vi "Draw.vi"(7 "menu in":refnum<class "menu.lvclass">, 8 "error in (no error)":errorcluster, 11 "text item in":refnum<class "text item.lvclass">) -> (0 "error out":errorcluster, 3 "text item out":refnum<class "text item.lvclass">)   [LabVIEW 2009, in "text item.lvclass"]
uses:
  text item.lvclass
  Menu/menu.lvclass
  text item.lvclass/text item.ctl
  ICON/icon.lvclass
  Text/text.lvclass
  Menu Item/menu item.lvclass
  Arrow/arrow.lvclass
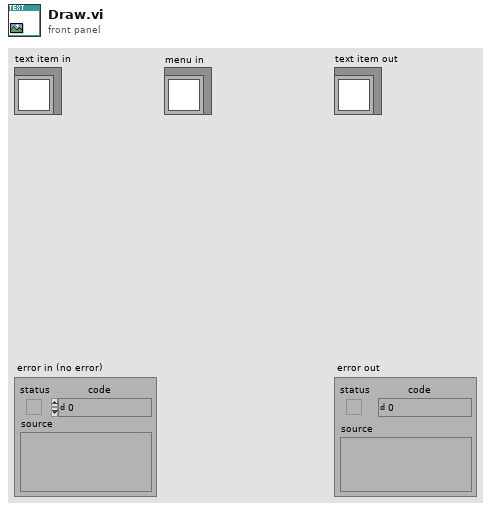
[diagram p1: front panel]
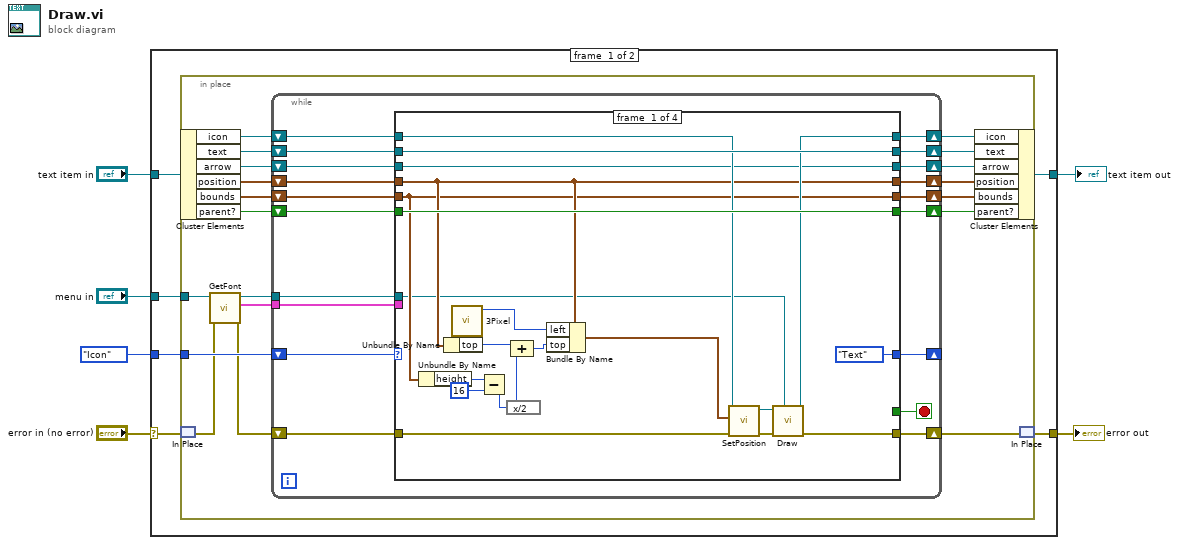
[diagram p0: block diagram]
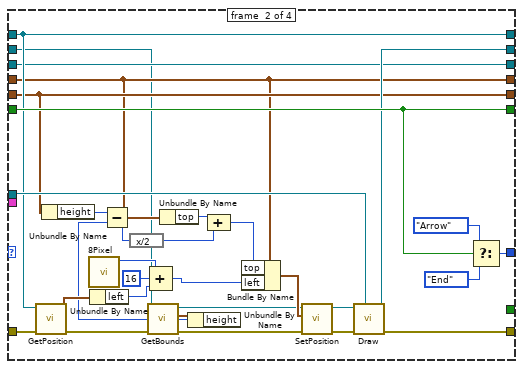
[diagram p2: hidden frame]
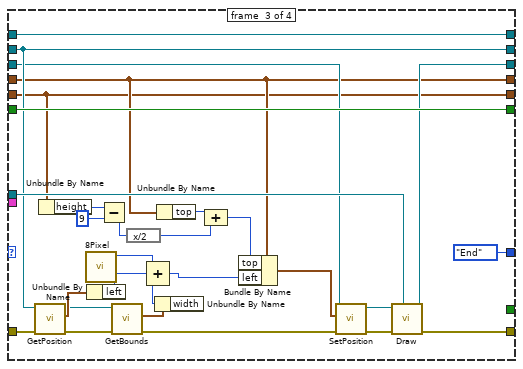
[diagram p3: hidden frame]
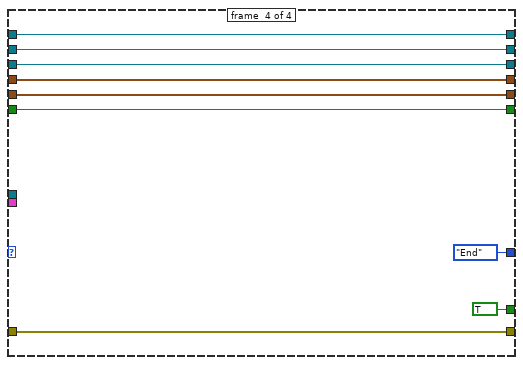
[diagram p4: hidden frame]
diagram:
  n1 = case shown="No Error" "error in (no error)" {
    selector: "error in (no error)" -> [w11 w142]
    tunnel: "text item in" -> [w12 w141]
    tunnel: [w10 w142] -> w4
    tunnel: [w9 w141] -> w3
    tunnel: "menu in" -> [w8 _]
    tunnel: enum16{"Icon", "Text", "Arrow", "End"}."Icon" -> [w7 _]
    frame #0 {
      n2 = in-place {
        in-place-border: w8 -> [w22]
        in-place-border: w7 -> [w31]
        n3 = in-place-cluster #1(w12) -> ("icon"=w30:refnum<class "icon.lvclass">, "text"=w29:refnum<class "text.lvclass">, "arrow"=w14:refnum<class "arrow.lvclass">, "position"=w28:cluster{"left":u32, "top":u32}, "bounds"=w27:cluster{"width":u32, "height":u32}, "parent?"=w16:bool)
        n4 = in-place-match #2(w11) -> (w20:errorcluster)
        n5 = call "GetFont.vi"("error in (no error)"=w20, "menu in"=w22) -> ("error out"=w19:errorcluster, "font"=w18:cluster{"name":string, "size":i16, "color":u32}, "menu out"=w21:refnum<class "menu.lvclass">)  [unwired: 7 in]
        n6 = while {
          shift-right: [w38] -> _
          shift-left: w31 -> [w50]
          shift-right: [w40] -> w17
          shift-left: w19 -> [w49]
          shift-right: [w41] -> w23
          shift-left: w27 -> [w45]
          shift-right: [w42] -> w24
          shift-left: w28 -> [w46]
          shift-right: [w43] -> w25
          shift-left: w29 -> [w47]
          shift-right: [w44] -> w26
          shift-left: w30 -> [w48]
          tunnel: w21 -> [w34]
          tunnel: w18 -> [w39]
          shift-right: [w37] -> w15
          shift-left: w16 -> [w36]
          shift-right: [w32] -> w13
          shift-left: w14 -> [w33]
          stop <- w35 stop-if-true
          n7 = case shown="\"Icon\"" w50 {
            tunnel: w49 -> [w66 w92 w125 w135]
            tunnel: w48 -> [w64 w93 w130 w140]
            tunnel: w47 -> [w70 w74 w124 w139]
            tunnel: w46 -> [w61 w82 w110 w138]
            tunnel: w45 -> [w60 w85 w109 w137]
            tunnel: [w63 w93 w130 w140] -> w44
            tunnel: [w70 w94 w124 w139] -> w43
            tunnel: [w61 w82 w110 w138] -> w42
            tunnel: [w60 w85 w109 w137] -> w41
            tunnel: [w65 w95 w115 w135] -> w40
            tunnel: w39 -> [_ _ _ _]
            tunnel: [enum16{"Icon", "Text", "Arrow", "End"}."Text" w100 enum16{"Icon", "Text", "Arrow", "End"}."End" enum16{"Icon", "Text", "Arrow", "End"}."End"] -> w38
            tunnel: [w71 w99 w131 w136] -> w37
            tunnel: w36 -> [w71 w99 w131 w136]
            tunnel: [_ _ _ TRUE] -> w35
            tunnel: w34 -> [w52 w96 w126 _]
            tunnel: w33 -> [w53 w80 w112 w132]
            tunnel: [w53 w80 w111 w132] -> w32
            frame #0 {
              n8 = Unbundle By Name(w60) -> ("height"=w58:u32)
              n9 = Unbundle By Name(w61) -> ("top"=w59:u32)
              n10 = call "3Pixel.vi"() -> ("3 pixel"=w51:u32)  [unwired: 11 in]
              n11 = Subtract(x=w58, y=u32 16) -> (x-y=w55:u32)
              n12 = expression code="x/2"(w55) -> (w54:u32)
              n13 = Compound Arithmetic op=ADD(w59, w54) -> (w56:u32)
              n14 = Bundle By Name(cluster=w61, "left"=w51, "top"=w56) -> (w62:cluster{"left":u32, "top":u32})
              n15 = call "SetPosition.vi"("error in (no error)"=w66, "position"=w62, "icon in"=w64) -> ("error out"=w67:errorcluster, "icon out"=w68:refnum<class "icon.lvclass">)  [unwired: 7 in]
              n16 = call "Draw.vi"("menu in"=w52, "error in (no error)"=w67, "icon in"=w68) -> ("error out"=w65:errorcluster, "icon out"=w63:refnum<class "icon.lvclass">)  [unwired: 7 in]
            }
            frame #1 {
              n17 = call "GetPosition.vi"("error in (no error)"=w92, "icon in"=w93) -> ("error out"=w79:errorcluster, "position"=w91:cluster{"left":u32, "top":u32})  [unwired: 7 in, 1 out]
              n18 = Unbundle By Name(w85) -> ("height"=w87:u32)
              n19 = call "8Pixel.vi"() -> ("8 pixel"=w88:u32)  [unwired: 11 in]
              n20 = Unbundle By Name(w91) -> ("left"=w73:u32)
              n21 = call "GetBounds.vi"("error in (no error)"=w79, "text in"=w74) -> ("error out"=w77:errorcluster, "bounds"=w76:cluster{"width":u32, "height":u32}, "text out"=w78:refnum<class "text.lvclass">)  [unwired: 7 in]
              n22 = Compound Arithmetic op=ADD(w88, u32 16 ("value"), w73) -> (w89:u32)
              n23 = Unbundle By Name(w82) -> ("top"=w83:u32)
              n24 = Unbundle By Name(w76) -> ("height"=w75:u32)
              n25 = Subtract(x=w87, y=w75) -> (x-y=w86:u32)
              n26 = expression code="x/2"(w86) -> (w84:u32)
              n27 = Compound Arithmetic op=ADD(w83, w84) -> (w81:u32)
              n28 = Bundle By Name(cluster=w82, "top"=w81, "left"=w89) -> (w90:cluster{"left":u32, "top":u32})
              n29 = call "SetPosition.vi"("error in (no error)"=w77, "position"=w90, "text in"=w78) -> ("error out"=w97:errorcluster, "text out"=w98:refnum<class "text.lvclass">)  [unwired: 7 in]
              n30 = call "Draw.vi"("menu in"=w96, "error in (no error)"=w97, "text in"=w98) -> ("error out"=w95:errorcluster, "text out"=w94:refnum<class "text.lvclass">)  [unwired: 7 in]
              n31 = Select(t=enum16{"Icon", "Text", "Arrow", "End"}."Arrow", s=w99, f=enum16{"Icon", "Text", "Arrow", "End"}."End") -> (s? t:f=w100:enum16{"Icon", "Text", "Arrow", "End"})
            }
            frame #2 {
              n32 = call "GetPosition.vi"("error in (no error)"=w125, "text in"=w124) -> ("error out"=w108:errorcluster, "position"=w113:cluster{"left":u32, "top":u32}, "text out"=w106:refnum<class "text.lvclass">)  [unwired: 7 in]
              n33 = Unbundle By Name(w109) -> ("height"=w121:u32)
              n34 = call "8Pixel.vi"() -> ("8 pixel"=w122:u32)  [unwired: 11 in]
              n35 = Unbundle By Name(w113) -> ("left"=w104:u32)
              n36 = Subtract(x=w121, y=u32 9) -> (x-y=w119:u32)
              n37 = call "GetBounds.vi"("error in (no error)"=w108, "text in"=w106) -> ("error out"=w107:errorcluster, "bounds"=w105:cluster{"width":u32, "height":u32})  [unwired: 7 in, 1 out]
              n38 = expression code="x/2"(w119) -> (w118:u32)
              n39 = Unbundle By Name(w105) -> ("width"=w103:u32)
              n40 = Compound Arithmetic op=ADD(w122, w104, w103) -> (w123:u32)
              n41 = Unbundle By Name(w110) -> ("top"=w117:u32)
              n42 = Compound Arithmetic op=ADD(w117, w118) -> (w116:u32)
              n43 = Bundle By Name(cluster=w110, "top"=w116, "left"=w123) -> (w114:cluster{"left":u32, "top":u32})
              n44 = call "SetPosition.vi"("error in (no error)"=w107, "position"=w114, "arrow in"=w112) -> ("error out"=w128:errorcluster, "arrow out"=w127:refnum<class "arrow.lvclass">)  [unwired: 7 in]
              n45 = call "Draw.vi"("menu in"=w126, "error in (no error)"=w128, "arrow in"=w127) -> ("error out"=w115:errorcluster, "arrow out"=w111:refnum<class "arrow.lvclass">)  [unwired: 7 in]
            }
            frame #3 {
            }
          }
        }
        n46 = in-place-cluster #1("icon"=w26, "text"=w25, "arrow"=w13, "position"=w24, "bounds"=w23, "parent?"=w15) -> (w9:refnum<class "text item.lvclass">)
        n47 = in-place-match #2(w17) -> (w10:errorcluster)
      }
    }
    frame #1 {
    }
  }
  "text item out" <- w3
  "error out" <- w4
